vi "FtpDirUpload.vi"(5 "アクティブ?(T)":bool=TRUE, 6 "パターン":string, 7 "FTP情報":T1={"FTPユーザ名"="", "FTPパスワード"="", "リモートディレクトリ"="/"}, 8 "Error In":errorcluster caption="エラー入力", 9 "ローカルディレクトリ":path, 10 "ポート番号 (21)":u16=21, 11 "ホスト名またはIPアドレス":string) -> (0 "Error Out":errorcluster caption="エラー出力")   [LabVIEW 2015]
uses:
  <vilib>/FTP/NI_FTP.lvlib
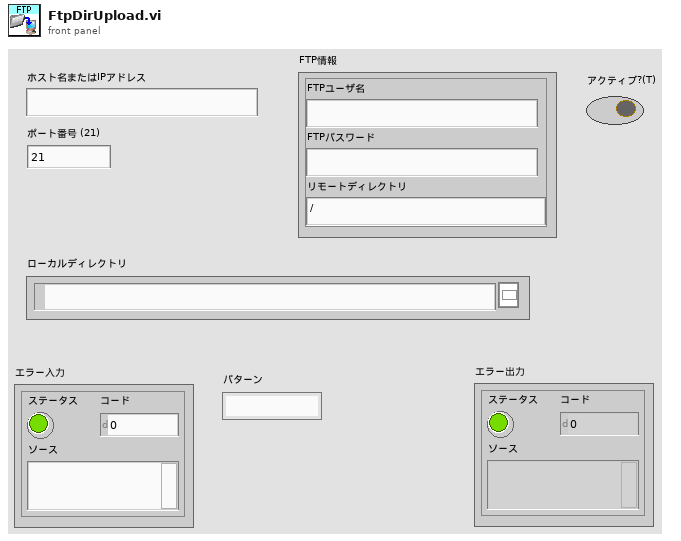
[diagram p1: front panel]
types:
  T1 = cluster{"FTPユーザ名":string, "FTPパスワード":string, "リモートディレクトリ":string}
  T2 = typedef "NI_FTP.lvlib/FTP Session.ctl" = refnum<k5>
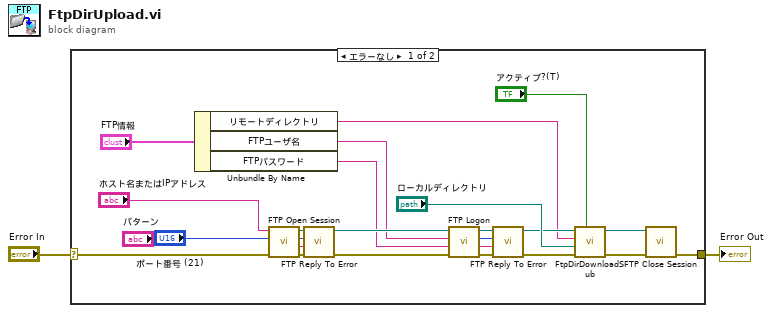
[diagram p0: block diagram]
diagram:
  n1 = case shown="エラーなし" "Error In" {
    selector: "Error In" -> [w11 w27]
    tunnel: [w7 w27] -> w1
    frame No Error {
      n2 = Unbundle By Name("FTP情報") -> ("リモートディレクトリ"=w5:string, "FTPユーザ名"=w4:string, "FTPパスワード"=w3:string)
      n3 = call <vilib>:"FTP Open Session.vi"("error in (no error)"=w11, "remote port (21)"="ポート番号 (21)", "address"="ホスト名またはIPアドレス") -> ("error out"=w14:errorcluster, "reply string"=w15:string, "reply code"=w16:i32, "ftp session"=w17:T2)  [unwired: 5 in]
      n4 = call <vilib>:"FTP Reply To Error.vi"("error in (no error)"=w14, "reply string in"=w15, "reply code in"=w16, "ftp session"=w17) -> ("error out"=w12:errorcluster, "ftp session out"=w13:T2)  [unwired: 2 out]
      n5 = call <vilib>:"FTP Logon.vi"("error in (no error)"=w12, "password"=w3, "user"=w4, "ftp session"=w13) -> ("error out"=w20:errorcluster, "reply string"=w21:string, "reply code"=w22:i32, "ftp session out"=w23:T2)  [unwired: 4 in]
      n6 = call <vilib>:"FTP Reply To Error.vi"("error in (no error)"=w20, "reply string in"=w21, "reply code in"=w22, "ftp session"=w23) -> ("error out"=w18:errorcluster, "ftp session out"=w19:T2)  [unwired: 2 out]
      n7 = call "FtpDirDownloadSub.vi"("アクティブ?(T)"="アクティブ?(T)", "error in (no error)"=w18, "ローカルディレクトリ"="ローカルディレクトリ", "directory path"=w5, "ftp session"=w19) -> ("error out"=w9:errorcluster, "ftp session out"=w10:T2)  [unwired: 5 in]
      n8 = call <vilib>:"FTP Close Session.vi"("error in (no error)"=w9, "ftp session"=w10) -> ("error out"=w7:errorcluster)  [unwired: 6 in, 3 out]
    }
    frame Error {
    }
  }
  "Error Out" <- w1
